vi "Quit Word.vi"(8 "error in (no error)":errorcluster, 11 "report in":refnum<class "NI_report.lvclass">) -> (0 "error out":errorcluster)   [LabVIEW 2024, in "LVarex.lvlib"]
uses:
  <vilib>/Utility/NIReport.llb/NI_report.lvclass
  LVarex.lvlib
  <vilib>/Utility/NIReport.llb/Word/NI_Word.lvclass
panel:
  # "Report Generation Close Report does not close the Word Session.\nThis VI gets an ActiveX handle to Word and invokes Quit."
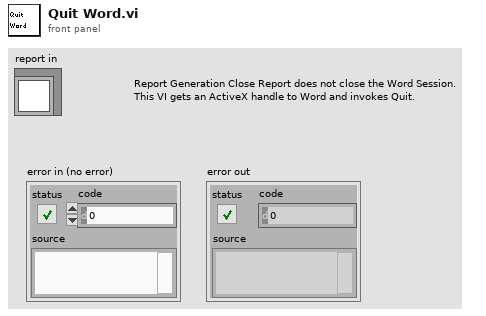
[diagram p1: front panel]
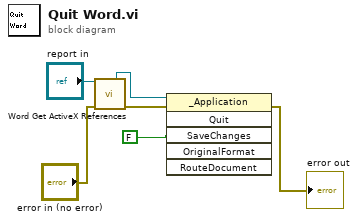
[diagram p0: block diagram]
diagram:
  n1 = call <vilib>:"Word Get ActiveX References.vi"("report in"="report in", "error in (no error)"="error in (no error)") -> ("Word._Application"=w5:refnum<k7>, "error out"=w3:errorcluster)  [unwired: 7 in, 5 out]
  n2 = invoke class="_Application" method="Quit"(reference=w5, error in=w3, "SaveChanges"=FALSE) -> (error out=→"error out":errorcluster)  [unwired: 3 in, 5 out]
